vi "Read Filter.vi"(7 "Channel (0: Channel A)":u16(ring) items=["Channel A", "Channel B"], 8 "error in (no error)":errorcluster, 11 "BH Druck PACE Series in":refnum<class "BH Druck PACE Series.lvclass">) -> (0 "error out":errorcluster, 1 "Filter Time Read (s)":dbl, 2 "Filter Band Read":dbl, 3 "BH Druck PACE Series out":refnum<class "BH Druck PACE Series.lvclass">, 4 "Filter Status":bool)   [LabVIEW 2022 SP3, in "BH Druck PACE Series.lvclass"]
uses:
  BH Druck PACE Series.lvclass
  BH Druck PACE Series.lvclass/BH Druck PACE Series.ctl
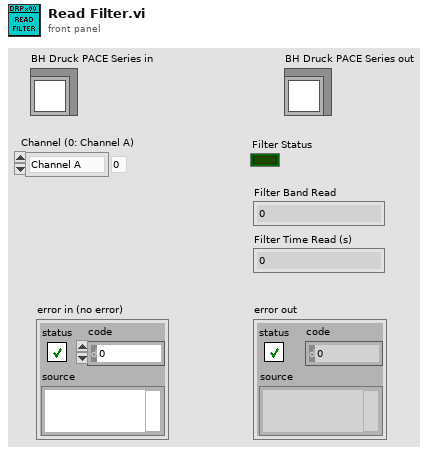
[diagram p1: front panel]
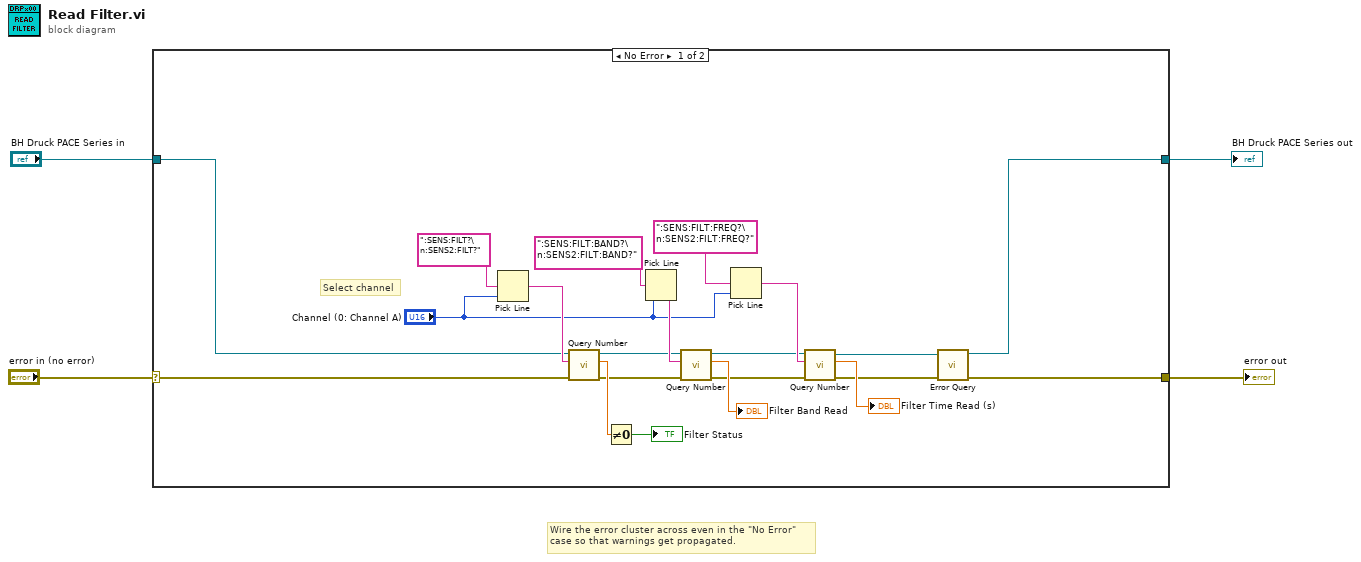
[diagram p0: block diagram]
diagram:
  # "Wire the error cluster across even in the \"No Error\"\ncase so that warnings get propagated."
  n1 = case shown="No Error" "error in (no error)" {
    selector: "error in (no error)" -> [w8 w27]
    tunnel: [w7 w27] -> w3
    tunnel: [w5 w26] -> w1
    tunnel: "BH Druck PACE Series in" -> [w6 w26]
    frame No Error {
      # "Select channel"
      n2 = Pick Line(multi-line string=":SENS:FILT?\n:SENS2:FILT?", line index="Channel (0: Channel A)") -> (output string=w23:string)  [unwired: 1 in]
      n3 = call-dynamic "Query Number.vi"("error in (no error)"=w8, "Query String"=w23, "BH Druck PACE Series in"=w6) -> ("error out"=w17:errorcluster, "Numeric Result"=w21:dbl, "BH Druck PACE Series out"=w14:refnum<class "BH Druck PACE Series.lvclass">)  [unwired: 6 in]
      n4 = Not Equal To 0?(x=w21) -> (x != 0?=→"Filter Status":bool)
      n5 = Pick Line(multi-line string=":SENS:FILT:BAND?\n:SENS2:FILT:BAND?", line index="Channel (0: Channel A)") -> (output string=w25:string)  [unwired: 1 in]
      n6 = call-dynamic "Query Number.vi"("error in (no error)"=w17, "Query String"=w25, "BH Druck PACE Series in"=w14) -> ("error out"=w16:errorcluster, "Numeric Result"=→"Filter Band Read":dbl, "BH Druck PACE Series out"=w13:refnum<class "BH Druck PACE Series.lvclass">)  [unwired: 6 in]
      n7 = Pick Line(multi-line string=":SENS:FILT:FREQ?\n:SENS2:FILT:FREQ?", line index="Channel (0: Channel A)") -> (output string=w20:string)  [unwired: 1 in]
      n8 = call-dynamic "Query Number.vi"("error in (no error)"=w16, "Query String"=w20, "BH Druck PACE Series in"=w13) -> ("error out"=w15:errorcluster, "Numeric Result"=→"Filter Time Read (s)":dbl, "BH Druck PACE Series out"=w12:refnum<class "BH Druck PACE Series.lvclass">)  [unwired: 6 in]
      n9 = call-dynamic "Error Query.vi"("error in (no error)"=w15, "BH Druck PACE Series in"=w12) -> ("error out"=w7:errorcluster, "BH Druck PACE Series out"=w5:refnum<class "BH Druck PACE Series.lvclass">)  [unwired: 8 in]
    }
    frame Error {
    }
  }
  "error out" <- w3
  "BH Druck PACE Series out" <- w1
